vi "ShortcutsTab-DeviceCMD.vi"(7 "DeviceData":T3) -> ()   [LabVIEW 2020]
uses:
  MainFrame/Queue/queue.ctl
  MainFrame/GlobalMainVI.vi
panel:
  out "KeyPress":string
  out "ScanCode":i16
  out "PlatMods":T1
  out "Run?":bool[](array[boolean])
  out "Array":T2(array[cluster])
  in  "Stop":bool
  out "Name":string
  out "CMD":T4
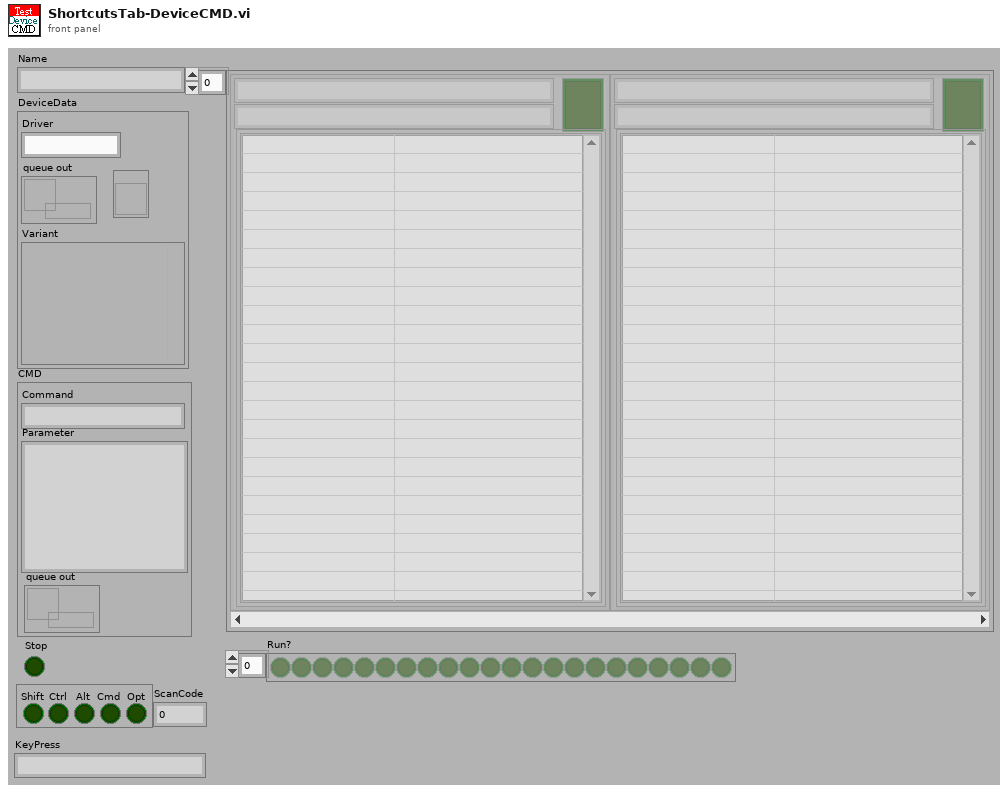
[diagram p1: front panel]
types:
  T1 = cluster{"Shift":bool, "Ctrl":bool, "Alt":bool, "Cmd":bool, "Opt":bool}
  T2 = cluster{"CronTabName":string, "Condition":string, cluster{"Script":string[][]}, "Enable?":bool}[]
  T3 = cluster{"Driver":string, "queue out":refnum<queue>, refnum<vi>, "Variant":variant}
  T4 = cluster{"Command":string, "Parameter":string, "queue out":refnum<queue>}
  T5 = typedef "queue.ctl" = enum16{"RT queue Init", "Module queue Init", "Recieve queue Init", "CMD EXE queue Init", "Get queue", "release all queue"}
  T6 = cluster{"CronTabName":string, "Condition":string, "Script":cluster{"Script":string[][]}, "Enable?":bool}
  T7 = enum16{"Init", "Add", "Enable", "Disable", "Get"}
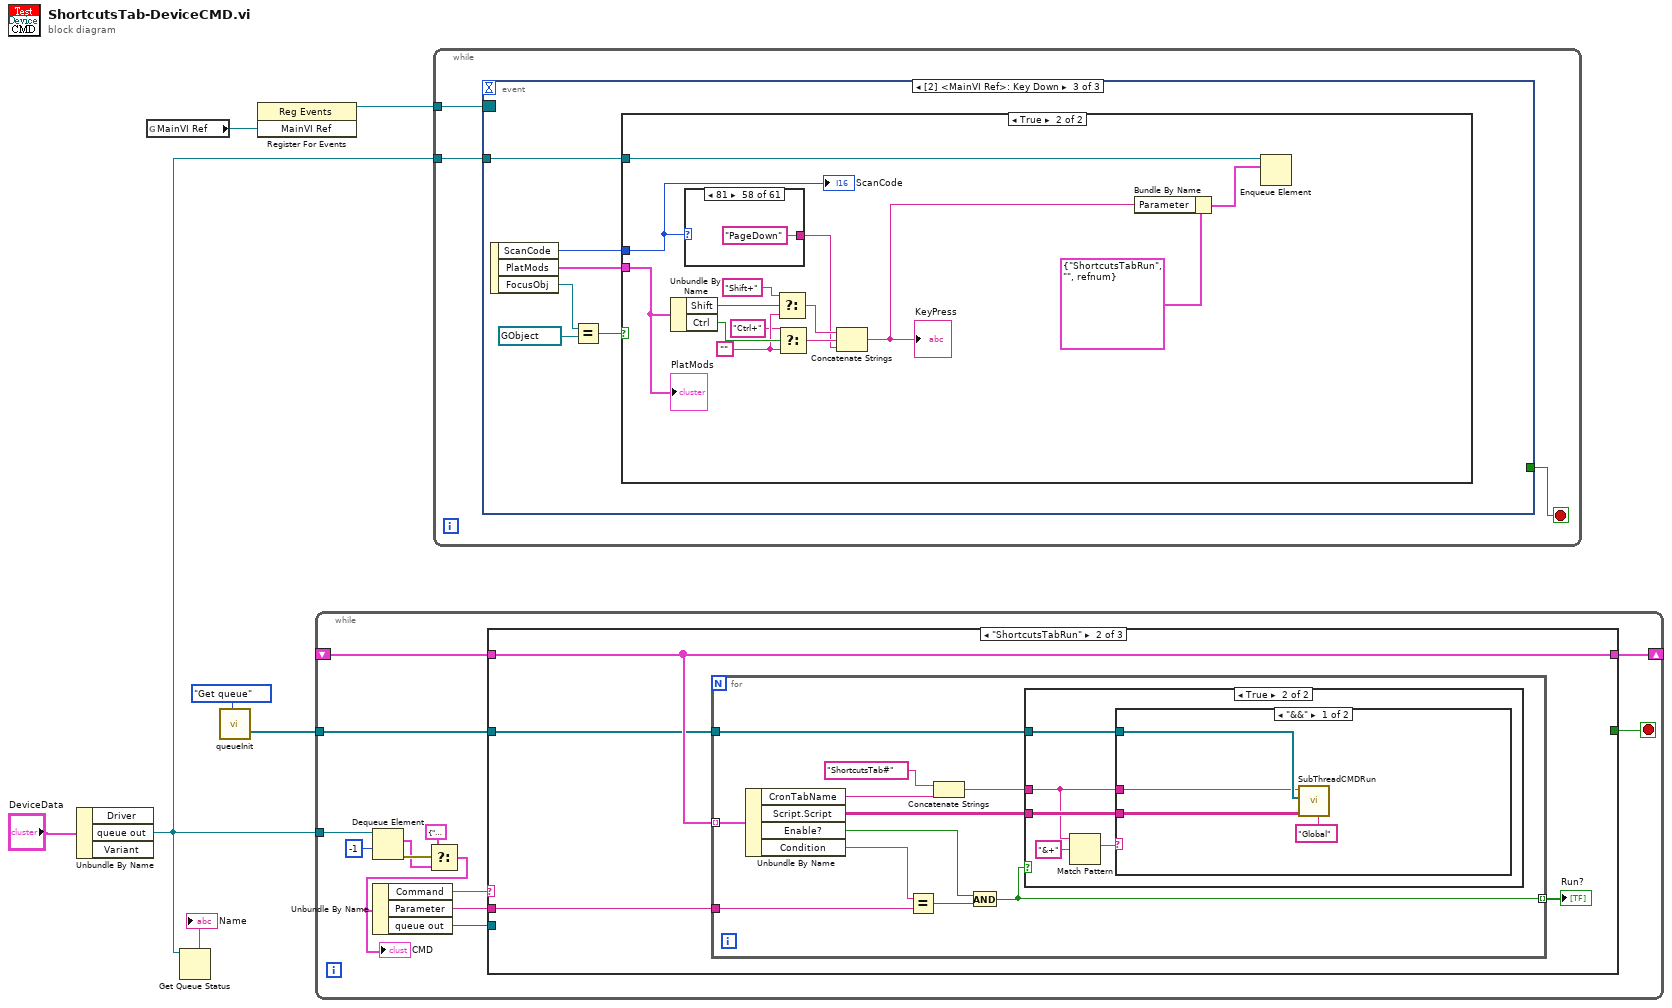
[diagram p0: block diagram]
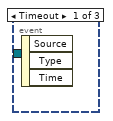
[diagram p2: hidden frame]
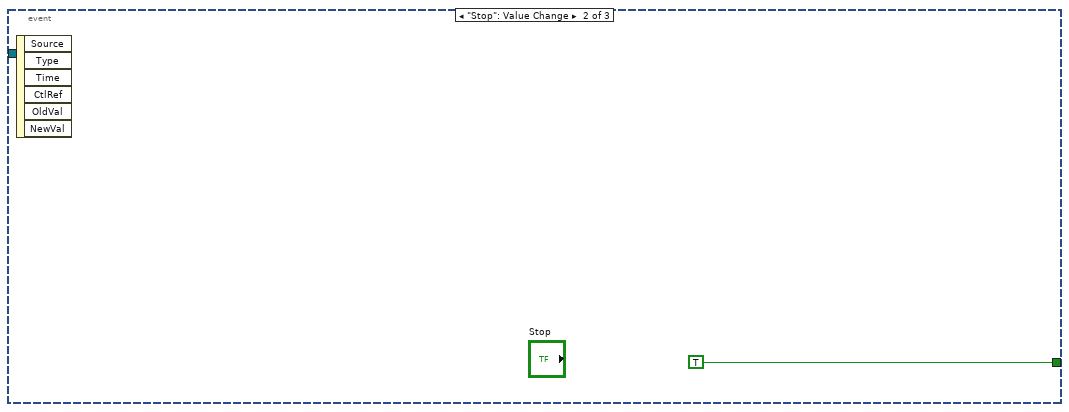
[diagram p3: hidden frame]
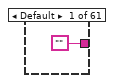
[diagram p5: hidden frame]
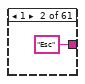
[diagram p6: hidden frame]
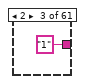
[diagram p7: hidden frame]
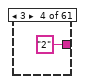
[diagram p8: hidden frame]
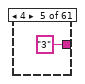
[diagram p9: hidden frame]
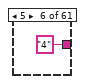
[diagram p10: hidden frame]
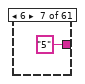
[diagram p11: hidden frame]
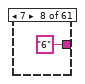
[diagram p12: hidden frame]
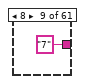
[diagram p13: hidden frame]
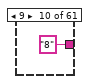
[diagram p14: hidden frame]
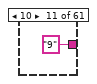
[diagram p15: hidden frame]
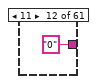
[diagram p16: hidden frame]
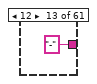
[diagram p17: hidden frame]
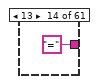
[diagram p18: hidden frame]
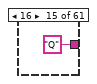
[diagram p19: hidden frame]
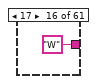
[diagram p20: hidden frame]
diagram:
  n1 = Unbundle By Name("DeviceData") -> ("queue out"=w5:refnum<queue>)  [unwired: 2 out]
  n2 = global read "GlobalMainVI.vi" "MainVI Ref"() -> (w2:refnum<vi>)
  n3 = Get Queue Status(queue=w5) -> (queue name=→"Name":string)  [unwired: 2 in, 7 out]
  n4 = call "queueInit.vi"("CMD"=queue."Get queue") -> ("CMD EXE thread queue"=w3:refnum<queue>[])  [unwired: 14 in, 4 out]
  n5 = register-events(w2) -> (reference out=w1:refnum<event-registration>)  [unwired: 2 in, 1 out]
  n6 = while {
    tunnel: w5 -> [w20]
    shift-right: [w10] -> _
    shift-left: _ -> [w9]
    tunnel: w3 -> [w8]
    stop <- w16 stop-if-true
    n7 = Dequeue Element(queue=w20, timeout in ms (-1)=-1) -> (element=w13:T4, error out=w14:errorcluster)  [unwired: 1 in, 2 out]
    n8 = Select(t=T4 {"Command"="Close", "Parameter"="", "queue out"=refnum}, s=w14, f=w13) -> (s? t:f=w12:T4)
    "CMD" <- w12
    n9 = Unbundle By Name(w12) -> ("Command"=w19:string, "Parameter"=w18:string, "queue out"=w17:refnum<queue>)
    n10 = case shown="\"ShortcutsTabRun\"" w19 {
      tunnel: w18 -> [_ w35 _]
      tunnel: w17 -> [_ _ _]
      tunnel: [_ _ w76] -> w16
      tunnel: [w22 w38 w77] -> w10
      tunnel: w9 -> [_ w38 w77]
      tunnel: w8 -> [_ w37 _]
      frame "ShortcutsTabUpdate", Default {
        n11 = call "ShortcutsTabNameIndex.vi"("OP"=T7."Get", "KeyTabName"="") -> ("KeyTableConditionS"=w23:string[], "Enable?S"=w24:bool[], "Scripts"=w25:cluster{"Script":string[][]}[], "KeyTabNameS"=w26:string[])  [unwired: 6 in]
        n12 = for {
          tunnel: w26 -> [w33] mode=indexing
          tunnel: w25 -> [w32] mode=indexing
          tunnel: w24 -> [w31] mode=indexing
          tunnel: w23 -> [w30] mode=indexing
          tunnel: [w29] -> w22 mode=indexing
          tunnel: T6 {"CronTabName"="", "Condition"="", "Script"={"Script"=[]}, "Enable?"=FALSE} ("Cluster") -> [w34]
          n13 = Bundle By Name(cluster=w34, "CronTabName"=w33, "Condition"=w30, "Script"=w32, "Enable?"=w31) -> (w29:T6)
        }
        "Array" <- w22
      }
      frame "ShortcutsTabRun" {
        n14 = for {
          tunnel: w38 -> [w49] mode=indexing
          tunnel: [w45] -> w36 mode=indexing
          tunnel: w37 -> [w44]
          tunnel: w35 -> [w39]
          n15 = Unbundle By Name(w49) -> ("CronTabName"=w48:string, "Script.Script"=w42:string[][], "Enable?"=w43:bool, "Condition"=w40:string)
          n16 = Equal?(x=w40, y=w39) -> (x = y?=w41:bool)
          n17 = Concatenate Strings("ShortcutsTab#" ("string"), w48) -> (w46:string)
          n18 = And(x=w43, y=w41) -> (x .and. y?=w45:bool)
          n19 = case shown="True" w45 {
            tunnel: w46 -> [_ w51]
            tunnel: w44 -> [_ w54]
            tunnel: w42 -> [_ w53]
            frame False {
            }
            frame True {
              n20 = Match Pattern(string=w51, regular expression="&+") -> (match substring=w50:string)  [unwired: 1 in, 3 out]
              n21 = case shown="\"&&\"" w50 {
                tunnel: w54 -> [w58 w65]
                tunnel: w53 -> [w57 w64]
                tunnel: w51 -> [w56 w59]
                frame "&&" {
                  n22 = call "SubThreadCMDRun.vi"("ID#CallBack"="Global", "Command"=w57, "Threads"=w58, "SubThreadName"=w56) -> ()  [unwired: 7 in, 1 out]
                }
                frame Default {
                  n23 = call "SubThreadNameIndex.vi"("SubThreadName"=w59) -> ("vi reference"=w63:refnum<vi>, "Find?"=w61:bool)  [unwired: 7 in, 2 out]
                  n24 = call "SubThreadCMDWait.vi"("vi reference"=w63) -> ("Run?"=w62:bool)  [unwired: 10 in]
                  n25 = And(x=w62, y=w61) -> (x .and. y?=w60:bool)
                  n26 = case shown="False" w60 {
                    tunnel: w65 -> [w69 _]
                    tunnel: w64 -> [w68 _]
                    tunnel: w59 -> [w67 w72]
                    frame False {
                      n27 = call "SubThreadCMDRun.vi"("ID#CallBack"="Global", "Command"=w68, "Threads"=w69, "SubThreadName"=w67) -> ()  [unwired: 7 in, 1 out]
                    }
                    frame True {
                      n28 = Match Pattern(string=w72, regular expression="#") -> (after substring=w70:string)  [unwired: 1 in, 3 out]
                      n29 = Concatenate Strings("CronTab: <", w70, "> is not finished before Crontab again!" ("string")) -> (w73:string)
                      n30 = call "SysLog.vi"("Mssage"=w73) -> ()  [unwired: 5 in]
                    }
                  }
                }
              }
            }
          }
        }
        "Run?" <- w36
      }
      frame "Close" {
        w76 = TRUE
        n31 = property on="Stop" class="Bool (strict)"("Val(Sgnl)"=w76) -> ()  [unwired: 2 in, 2 out]
      }
    }
  }
  n32 = while {
    tunnel: w5 -> [w78]
    tunnel: w1 -> [w79]
    stop <- w80 stop-if-true
    n33 = event shown="[2] <MainVI Ref>: Key Down" {
      selector: w79 -> [_ _ _]
      dyn-events: _ -> [_ _ _]
      timeout: _ -> [_ _ _]
      tunnel: [_ TRUE ("Stop") _] -> w80
      tunnel: w78 -> [_ _ w82]
      event Timeout {
        n34 = event-data() -> ()  [unwired: 1 in, 3 out]
      }
      event "Stop": Value Change {
        n35 = event-data() -> ()  [unwired: 1 in, 6 out]
      }
      event Key Down {
        n36 = event-data() -> ("ScanCode"=w86:i16, "PlatMods"=w87:T1, "FocusObj"=w84:refnum<vi>)  [unwired: 1 in]
        n37 = Equal?(x=w84, y=refnum<vi> refnum ("FocusObj")) -> (x = y?=w85:bool)
        n38 = case shown="True" w85 {
          tunnel: w87 -> [_ w101]
          tunnel: w86 -> [_ w93]
          tunnel: w82 -> [_ w91]
          frame False {
          }
          frame True {
            w97 = ""
            n39 = Unbundle By Name(w101) -> ("Shift"=w100:bool, "Ctrl"=w98:bool)
            n40 = case shown="81" w93 {
              tunnel: ["" "Esc" "1" "2" "3" "4" "5" "6" "7" "8" "9" "0" "-" "=" "Q" "W" "E" "R" "T" "Y" "U" "I" "O" "P" "[" "]" "]" "A" "S" "D" "F" "G" "H" "J" "L" "Z" "X" "C" "V" "B" "N" "M" "<" ">" "?" "F2" "F3" "F4" "F5" "F6" "F7" "F8" "F9" "F10" "Home" "PageUp" "End" "PageDown" "Del" "F11" "F12"] -> w92
              frame Default {
              }
              frame 1 {
              }
              frame 2 {
              }
              frame 3 {
              }
              frame 4 {
              }
              frame 5 {
              }
              frame 6 {
              }
              frame 7 {
              }
              frame 8 {
              }
              frame 9 {
              }
              frame 10 {
              }
              frame 11 {
              }
              frame 12 {
              }
              frame 13 {
              }
              frame 16 {
              }
              frame 17 {
              }
              frame 18 {
              }
              frame 19 {
              }
              frame 20 {
              }
              frame 21 {
              }
              frame 22 {
              }
              frame 23 {
              }
              frame 24 {
              }
              frame 25 {
              }
              frame 26 {
              }
              frame 27 {
              }
              frame 28 {
              }
              frame 30 {
              }
              frame 31 {
              }
              frame 32 {
              }
              frame 33 {
              }
              frame 34 {
              }
              frame 35 {
              }
              frame 36 {
              }
              frame 37 {
              }
              frame 44 {
              }
              frame 45 {
              }
              frame 46 {
              }
              frame 47 {
              }
              frame 48 {
              }
              frame 49 {
              }
              frame 50 {
              }
              frame 51 {
              }
              frame 52 {
              }
              frame 53 {
              }
              frame 60 {
              }
              frame 61 {
              }
              frame 62 {
              }
              frame 63 {
              }
              frame 64 {
              }
              frame 65 {
              }
              frame 66 {
              }
              frame 67 {
              }
              frame 68 {
              }
              frame 71 {
              }
              frame 73 {
              }
              frame 79 {
              }
              frame 81 {
              }
              frame 83 {
              }
              frame 87 {
              }
              frame 88 {
              }
            }
            n41 = Select(t="Shift+", s=w100, f=w97) -> (s? t:f=w95:string)
            n42 = Select(t="Ctrl+", s=w98, f=w97) -> (s? t:f=w94:string)
            n43 = Concatenate Strings(w95, w94, w92) -> (w89:string)
            "KeyPress" <- w89
            n44 = Bundle By Name(cluster=T4 {"Command"="ShortcutsTabRun", "Parameter"="", "queue out"=refnum} ("element"), "Parameter"=w89) -> (w88:T4)
            n45 = Enqueue Element(queue=w91, element=w88) -> ()  [unwired: 2 in, 3 out]
            "PlatMods" <- w101
            "ScanCode" <- w93
          }
        }
      }
    }
  }
